vi "Global Vairable.vi"() -> ()   [LabVIEW 2015]
panel:
  out "auto close":bool
  out "exit":bool
  out "Calibrated":bool
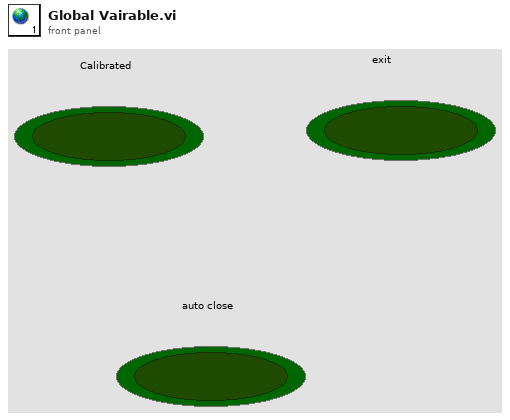
[diagram p1: front panel]
diagram:
